vi "Diagonal 2 Jacobian Matrix.vi"(10 "Jacobian Diagonal Out":dbl[](array[numeric])) -> (2 "Stiffness Jacobian In":T1=[[1000000.0, 0.0, 0.0, 0.0, 0.0, 0.0], [0.0, 1000000.0, 0.0, 0.0, 0.0, 0.0], [0.0, 0.0, 1000000.0, 0.0, 0.0, 0.0], [0.0, 0.0, 0.0, 1000000.0, 0.0, 0.0], [0.0, 0.0, 0.0, 0.0, 1000000.0, 0.0], [0.0, 0.0, 0.0, 0.0, 0.0, 1000000.0]])   [LabVIEW 2013]
uses:
  Stiffness Matrix.ctl
panel:
  # "dDx"
  # "dDy"
  # "dDz"
  # "dRx"
  # "dRy"
  # "dRz"
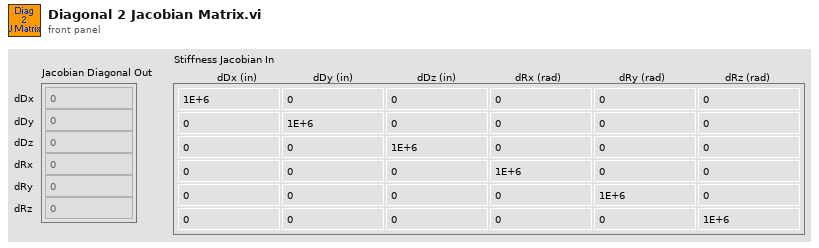
[diagram p1: front panel]
types:
  T1 = typedef "Stiffness Matrix.ctl" = dbl[][]
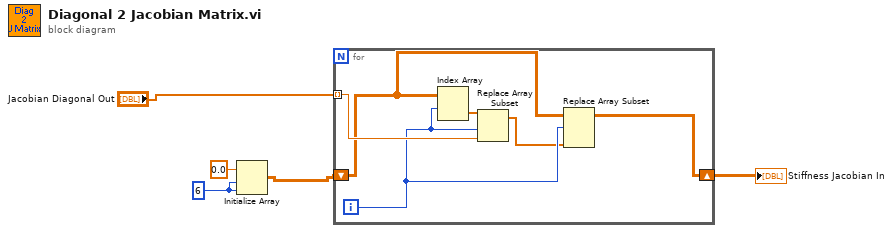
[diagram p0: block diagram]
diagram:
  w3 = 6 ("dimension size")
  n1 = Initialize Array(0.0 ("element"), w3, w3) -> (w2:dbl[][])
  n2 = for {
    tunnel: "Jacobian Diagonal Out" -> [w10] mode=indexing
    shift-right: [w6] -> w1
    shift-left: w2 -> [w9]
    i -> [w8]
    n3 = Index Array(array=w9, index (row)=w8) -> (element=w11:dbl[])  [unwired: 1 in]
    n4 = Replace Array Subset(array=w11, new element=w10, index=w8) -> (w7:dbl[])
    n5 = Replace Array Subset(array=w9, new element=w7, index (row)=w8) -> (w6:dbl[][])  [unwired: 1 in]
  }
  "Stiffness Jacobian In" <- w1
